vi "Construct Protected Connection Writer.vi"(11 "Connection Reference":refnum<data-value>) -> (3 "ProtectedConnectionWriter out":refnum<class "ProtectedConnectionWriter.lvclass">)   [LabVIEW 2020, in "ProtectedConnectionWriter.lvclass"]
uses:
  <vilib>/gpm_packages/@cs/Network-interface/Source/ProtectedConnectionWriter/ProtectedConnectionWriter.lvclass
  <vilib>/gpm_packages/@cs/Network-interface/Source/Connection Reference/Connection Reference/Connection Reference.lvclass
  <vilib>/gpm_packages/@cs/Network-interface/Source/ProtectedConnectionWriter/ProtectedConnectionWriter.lvclass/ProtectedConnectionWriter.ctl
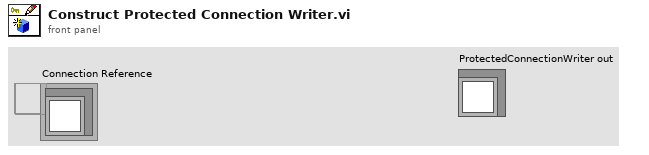
[diagram p1: front panel]
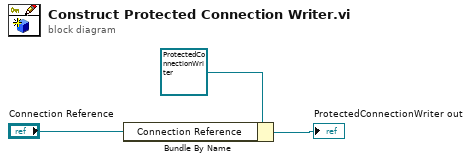
[diagram p0: block diagram]
diagram:
  n1 = Bundle By Name(cluster=refnum<class "ProtectedConnectionWriter.lvclass"> refnum ("ProtectedConnectionWriter in"), "Connection Reference"="Connection Reference") -> (→"ProtectedConnectionWriter out":refnum<class "ProtectedConnectionWriter.lvclass">)
